vi "Stop Core.vi"(10 "final error code":i32, 11 "Data Repository in":refnum<class "Data Repository.lvclass">) -> (3 "Data Repository out":refnum<class "Data Repository.lvclass">)   [LabVIEW 2020, in "Data Repository.lvlib" / "Data Repository.lvclass"]
doc: "(<B>Filename</B>: Actor Framework.lvlib:Actor.lvclass:Stop Core.vi)\n\nDefines what the actor does before it stops. Use the <B>final error code</B> input to determine whether the actor shut down in response to an error.\n\nThis implementation releases all the notifiers obtained by the Data Repository."
uses:
  Data Repository.lvclass
  PPL/HDH.Data.Generic.lvlibp/Synchronization/Notifier/Notifier.lvclass
  Data Repository.lvclass/Data Repository.ctl
  PPL/HDH.Actor Framework.Core.Actor.lvlibp/1abvi3w/vi.lib/ActorFramework/Actor/Actor.lvclass
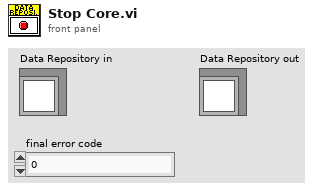
[diagram p1: front panel]
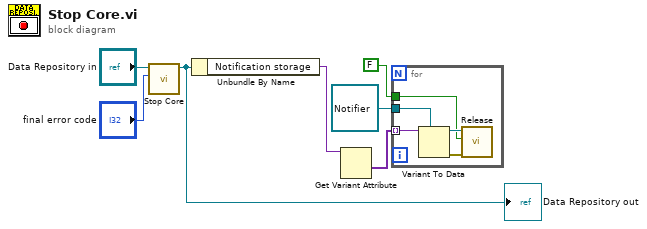
[diagram p0: block diagram]
diagram:
  n1 = call-parent "Stop Core.vi"("final error code"="final error code", "Actor in"="Data Repository in") -> ("Actor out"=w5:refnum<class "Data Repository.lvclass">)  [unwired: 9 in]
  "Data Repository out" <- w5
  n2 = Unbundle By Name(w5) -> ("Notification storage"=w4:variant)
  n3 = Get Variant Attribute(Variant=w4) -> (values=w1:variant[])  [unwired: 3 in, 3 out]
  n4 = for {
    tunnel: w1 -> [w12] mode=indexing
    tunnel: refnum<class "Notifier.lvclass"> refnum ("HDH.Data.Generic.lvlibp:Notifier.lvclass") -> [w11]
    tunnel: FALSE ("Force destroy? (F)") -> [w8]
    n5 = Variant To Data(type=w11, Variant=w12) -> (data=w10:refnum<class "Notifier.lvclass">, error out=w9:errorcluster)  [unwired: 1 in]
    n6 = call "Release.vi"("error in (no error)"=w9, "Force destroy? (F)"=w8, "Notifier in"=w10) -> ()  [unwired: 6 in, 3 out]
  }
